vi "DSF.Engine.Memory.Index FIFO.Destroy.vi"(8 "error in (no error)":errorcluster, 11 "Index FIFO in":refnum<class "DSF.Engine.Memory.Index FIFO.lvclass">) -> (0 "error out":errorcluster)   [LabVIEW 2016, in "DSF.Engine.lvlib" / "DSF.Engine.Memory.Index FIFO.lvclass"]
uses:
  DSF.Engine.Memory.Index FIFO.lvclass
  DSF.Engine.Memory.Index FIFO.lvclass/DSF.Engine.Memory.Index FIFO.ctl
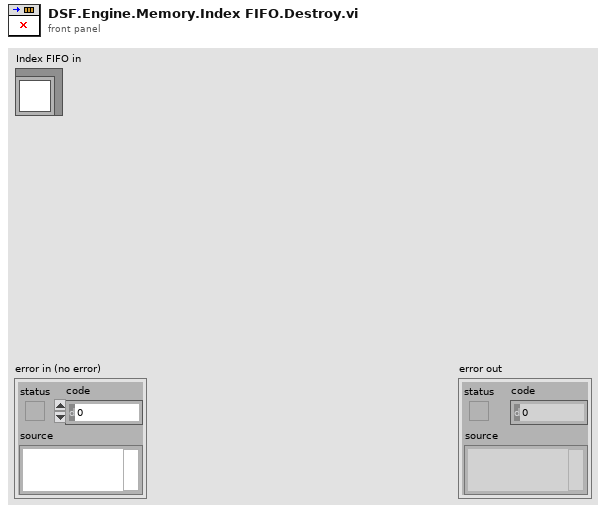
[diagram p1: front panel]
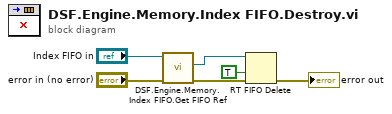
[diagram p0: block diagram]
diagram:
  n1 = call "DSF.Engine.Memory.Index FIFO.Get FIFO Ref.vi"("error in (no error)"="error in (no error)", "Index FIFO in"="Index FIFO in") -> ("error out"=w3:errorcluster, "FIFO"=w2:refnum<k33>)  [unwired: 7 in, 1 out]
  n2 = RT FIFO Delete(0:w2, 2:TRUE ("force destroy? (F)"), 3:w3) -> (11:→"error out":errorcluster)
